vi "Array to U64.vi"(7 "Input Array I16":i16[](array[numeric])=[0, 0, 0, 0]) -> (8 "Output U64":u64)   [LabVIEW 2014]
panel:
  # "Copyright 2014 Vidrio Technologies\nScanImage 5 software is licensed under the Apache License, Version 2.0 (the \"License\"); you may not use any files contained\nwithin the ScanImage 5 release except in compliance with the License. You may obtain a copy of the License at\n http://www.apache.org/licenses/LICENSE-2.0\nUnless required by applicable law or agreed to in writing, software distributed under the License is distributed on an\n\"AS IS\" BASIS, WITHOUT WARRANTIES OR CONDITIONS OF ANY KIND, either express or implied. See the License for the\n specific language governing permissions and limitations under the License."
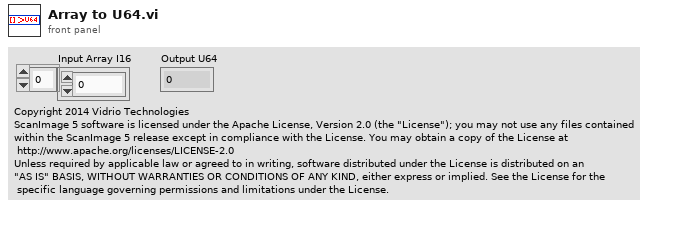
[diagram p1: front panel]
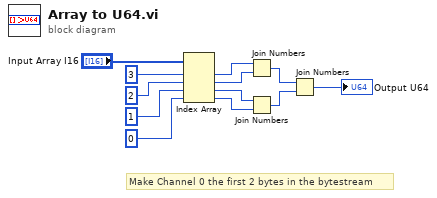
[diagram p0: block diagram]
diagram:
  # "Make Channel 0 the first 2 bytes in the bytestream"
  n1 = Index Array(array="Input Array I16", index #1=3 ("index"), index #2=2 ("index"), index #3=1 ("index"), index #4=0 ("index")) -> (element #1=w11:i16, element #2=w10:i16, element #3=w9:i16, element #4=w8:i16)
  n2 = Join Numbers(hi=w11, lo=w10) -> ((hi.lo)=w7:u32)
  n3 = Join Numbers(hi=w9, lo=w8) -> ((hi.lo)=w6:u32)
  n4 = Join Numbers(hi=w7, lo=w6) -> ((hi.lo)=→"Output U64":u64)
